vi "Test GUID.vi"() -> ()   [LabVIEW 2021]
uses:
  DataTypes_CIF_U.lvlib
panel:
  out "Pass":bool
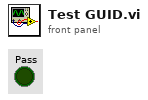
[diagram p1: front panel]
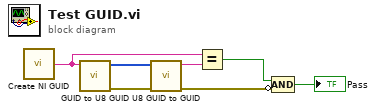
[diagram p0: block diagram]
diagram:
  n1 = call <vilib>:"Create NI GUID.vi"() -> ("NI GUID"=w3:string)
  n2 = call "GUID to U8 GUID.vi"("GUID In"=w3) -> ("error out"=w5:errorcluster, "U8 GUID"=w6:u8[])  [unwired: 9 in]
  n3 = call "U8 GUID to GUID.vi"("error in (no error)"=w5, "U8 GUID"=w6) -> ("error out"=w1:errorcluster, "GUID In"=w4:string)  [unwired: 8 in]
  n4 = Equal?(x=w3, y=w4) -> (x = y?=w2:bool)
  n5 = Compound Arithmetic op=AND(w2, invert w1) -> (→"Pass":bool)
